vi "configure generador FULL.vi"(8 "error in":errorcluster, 10 "Config Pulse":T1={"Channel"=0, "Frequency"=0.0, "Width Time"=0.0, "Amplitude"=0.0, "DC Offset"=0.0, "Load"=0.0, "Leading Edge Time"=0.0, "Trailing Edge Time"=0.0, "Delay"=0.0, "Out"=FALSE, "/Out"=FALSE, "Trigger Level Sync"=0, "Trigger Sync Out"=0, "Vasic Theorical"=50.0} {"Vasic Theorical" min=1.0 max=1000000.0 step=1.0 format="%#_6pV"; "Frequency" min=0.001 max=333000000.0 step=1000.0 format="%#_6pHz"; "Leading Edge Time" min=1e-09 max=1.0 step=1e-10 format="%#_6ps"; "Trailing Edge Time" min=1e-09 max=1.0 step=1e-10 format="%#_6ps"; "Delay" min=0.0 max=1.0 step=1e-12 format="%#_6ps"; "Trigger Level Sync" items=["ECL", "TTL"]; "Trigger Sync Out" items=["AB"=3, "B"=2, "A"=1, "None"=0]; "Load" min=1.0 max=1000000.0 step=1.0 format="%#_6p"; "DC Offset" min=-10.0 max=10.0 step=0.1 format="%#_6pV"; "Amplitude" min=0.05 max=5.0 step=0.001 format="%#_6pV"; "Width Time" min=1.5e-09 max=1.0 step=1e-10 format="%#_6ps"; "Channel" items=["Channel1"=1, "Channel2"=2]}, 11 "VISA Key 81160A":refnum<visa-resource-name>) -> (0 "error out":errorcluster, 2 "Amplitude":dbl, 3 "VISA Key 81160A 2":refnum<visa-resource-name>)   [LabVIEW 2019]
uses:
  GenPulse_configurar.ctl
  Viejos/Alfredo LABVIEW/Set-up verificador ASICs/Lib Agilent 81160A/Agilent 81150/Agilent 81150.lvlib
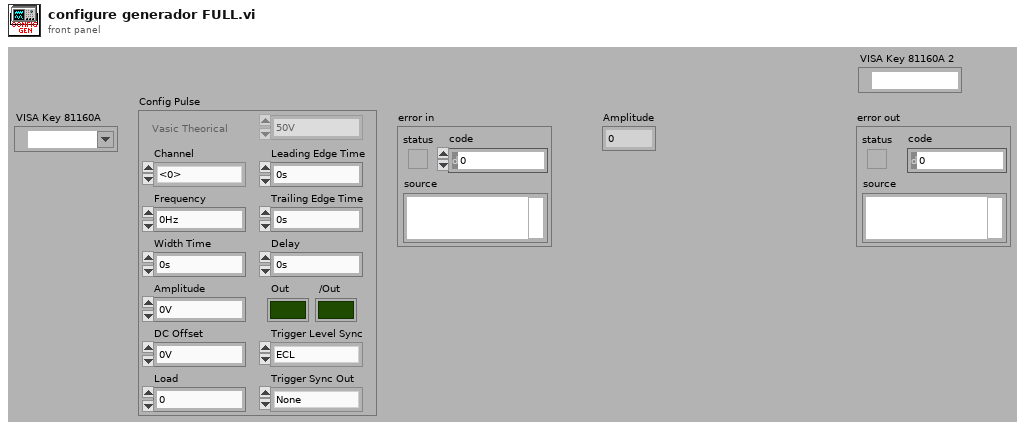
[diagram p1: front panel]
types:
  T1 = typedef "GenPulse_configurar.ctl" = cluster{"Channel":u16, "Frequency":dbl, "Width Time":dbl, "Amplitude":dbl, "DC Offset":dbl, "Load":dbl, "Leading Edge Time":dbl, "Trailing Edge Time":dbl, "Delay":dbl, "Out":bool, "/Out":bool, "Trigger Level Sync":u16, "Trigger Sync Out":u16, "Vasic Theorical":dbl}
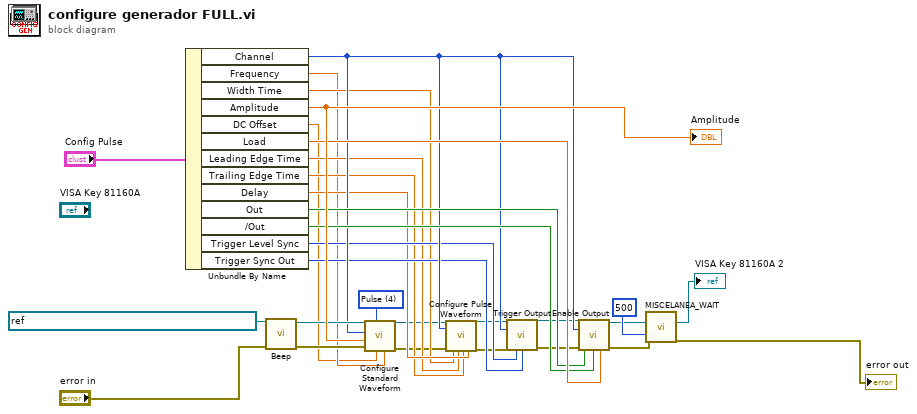
[diagram p0: block diagram]
diagram:
  w5 = u16 4 items=["Sine", "Square", "Ramp Up", "Ramp Down", "Pulse", "Noise", "DC"] ("Waveform (0: Sine)")
  n1 = Unbundle By Name("Config Pulse") -> ("Channel"=w20:u16, "Frequency"=w7:dbl, "Width Time"=w10:dbl, "Amplitude"=w29:dbl, "DC Offset"=w6:dbl, "Load"=w23:dbl, "Leading Edge Time"=w11:dbl, "Trailing Edge Time"=w12:dbl, "Delay"=w13:dbl, "Out"=w21:bool, "/Out"=w22:bool, "Trigger Level Sync"=w16:u16, "Trigger Sync Out"=w17:u16)
  "Amplitude" <- w29
  n2 = call "Beep.vi"("VISA resource name"=refnum<visa-resource-name> "USB0::0x0957::0x4108::MY51400682::INSTR", "error in (no error)"="error in") -> ("VISA resource name out"=w26:refnum<visa-resource-name>, "error out"=w25:errorcluster)  [unwired: 12 in]
  n3 = call "Configure Standard Waveform.vi"("Frequency (1000.0 Hz)"=w7, "DC Offset (0.0 Volts)"=w6, "Waveform (0: Sine)"=w5, "error in (no error)"=w25, "Amplitude (1.0 Vpp)"=w29, "Channel (1: Channel1)"=w20, "VISA resource name"=w26) -> ("error out"=w9:errorcluster, "VISA resource name out"=w8:refnum<visa-resource-name>)  [unwired: 3 in]
  n4 = call "Configure Pulse Waveform.vi"("VISA resource name"=w8, "Channel (1: Channel1)"=w20, "error in (no error)"=w9, "Width (1.5E-9 Sec)"=w10, "Leading Edge Time\n(1.0E-9 Sec)"=w11, "Trailing Edge Time\n(1.0E-9 Sec)"=w12, "Delay\n(0.0 Seconds)"=w13) -> ("VISA resource name out"=w14:refnum<visa-resource-name>, "error out"=w15:errorcluster)  [unwired: 11 in]
  n5 = call "Trigger Output.vi"("VISA resource name"=w14, "Channel (1: Channel1)"=w20, "error in (no error)"=w15, "Trigger Sync Out (1: A)"=w16, "Trigger Level Sync (0: ECL)"=w17) -> ("VISA resource name out"=w18:refnum<visa-resource-name>, "error out"=w19:errorcluster)  [unwired: 9 in]
  n6 = call "Enable Output.vi"("VISA resource name"=w18, "Channel (1: Channel1)"=w20, "error in (no error)"=w19, "Enable Output (T: Enable)"=w21, "Enable Output Complement (T: Enable)"=w22, "Load (50 Ohm)"=w23) -> ("VISA resource name out"=→"VISA Key 81160A 2":refnum<visa-resource-name>, "error out"=w27:errorcluster)  [unwired: 8 in]
  n7 = call "MISCELANEA_WAIT.vi"("ms wait IN"=u32 500, "Error IN"=w27) -> ("Error OUT"=→"error out":errorcluster)  [unwired: 16 in, 1 out]
